vi "Empty Block Diagram.vi"(8 "error in (no error)":errorcluster, 11 "VI in":refnum<vi>) -> (0 "error out":errorcluster, 3 "reference out":refnum<vi>)   [LabVIEW 2020, in "Mock Class Generator.lvclass"]
uses:
  Mock Class Generator.lvclass
  <vilib>/Utility/traverseref.llb/TRef TravTarget.ctl
  <vilib>/Utility/traverseref.llb/VI Scripting - Traverse.lvlib
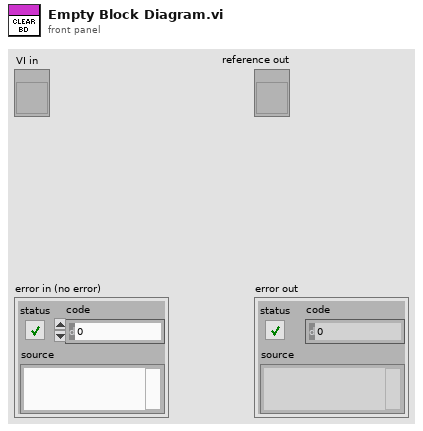
[diagram p1: front panel]
types:
  T1 = typedef "TRef TravTarget.ctl" = enum16{"FP", "BD", "Other"}
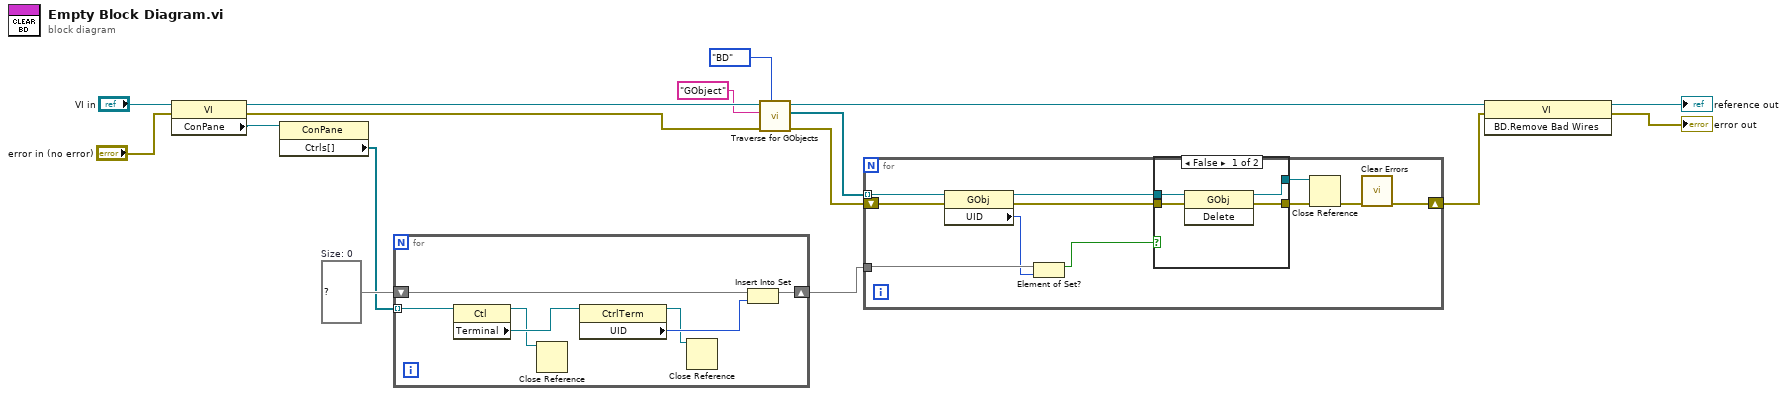
[diagram p0: block diagram]
diagram:
  w3 = set{i32} {}  # Size: 0
  n1 = property class="VI"(reference="VI in", error in="error in (no error)") -> (reference out=w13:refnum<vi>, error out=w12:errorcluster, "ConPane"=w4:refnum<vi>)
  n2 = property class="ConPane"(reference=w4) -> ("Ctrls[]"=w2:refnum<vi>[])  [unwired: 1 in, 2 out]
  n3 = for {
    shift-right: [w21] -> w1
    shift-left: w3 -> [w23]
    tunnel: w2 -> [w22] mode=indexing
    n4 = property class="Ctl"(reference=w22) -> (reference out=w17:refnum<vi>, "Terminal"=w18:refnum<vi>)  [unwired: 1 in, 1 out]
    n5 = Close Reference(reference=w17) -> ()  [unwired: 1 in, 1 out]
    n6 = property class="CtrlTerm"(reference=w18) -> (reference out=w19:refnum<vi>, "UID"=w20:i32)  [unwired: 1 in, 1 out]
    n7 = Close Reference(reference=w19) -> ()  [unwired: 1 in, 1 out]
    n8 = Insert Into Set(10:w20, 11:w23) -> (3:w21:set{i32})  [unwired: 1 out]
  }
  n9 = call <vilib>:"Traverse for GObjects.vi"("Traverse Target"=TRef_TravTarget."BD", "error in (no error)"=w12, "Class Name"="GObject", "VI Refnum"=w13) -> ("error out"=w11:errorcluster, "References"=w9:refnum<vi>[], "dup VI Refnum"=w7:refnum<vi>)  [unwired: 4 in, 1 out]
  n10 = for {
    tunnel: w9 -> [w26] mode=indexing
    shift-right: [w33] -> w5
    shift-left: w11 -> [w30]
    tunnel: w1 -> [w29]
    n11 = property class="GObj"(reference=w26, error in=w30) -> (reference out=w25:refnum<vi>, error out=w27:errorcluster, "UID"=w24:i32)
    n12 = Element of Set?(10:w24, 11:w29) -> (3:w28:bool)
    n13 = case shown="False" w28 {
      tunnel: [w38 w39] -> w34
      tunnel: [w37 w40] -> w31
      tunnel: w27 -> [w36 w39]
      tunnel: w25 -> [w35 w40]
      frame False {
        n14 = invoke class="GObj" method="Delete"(reference=w35, error in=w36) -> (reference out=w37:refnum<vi>, error out=w38:errorcluster)  [unwired: 1 in, 1 out]
      }
      frame True {
      }
    }
    n15 = Close Reference(reference=w31, error in (no error)=w34) -> (error out=w32:errorcluster)
    n16 = call <vilib>:"Clear Errors.vi"("error in (no error)"=w32) -> ("error out"=w33:errorcluster)  [unwired: 5 in, 1 out]
  }
  n17 = invoke class="VI" method="BD.Remove Bad Wires"(reference=w7, error in=w5) -> (reference out=→"reference out":refnum<vi>, error out=→"error out":errorcluster)  [unwired: 1 in, 1 out]
